vi "Proceed.vi"(7 "component is ready (Y)":bool=TRUE, 8 "error in (no error)":errorcluster, 10 "ProceedMessage":refnum<class "ProceedMessage.lvclass">, 11 "DAQCascade512II in":refnum<class "DAQCascade512II.lvclass">) -> (0 "error out":errorcluster, 2 "all observers are ready?":bool, 3 "DAQCascade512II out":refnum<class "DAQCascade512II.lvclass">)   [LabVIEW 2012, in "DAQCascade512II.lvclass"]
doc: "The Proceed method is used to check if your component is ready. Also it checks if the observers are ready. When the observers and the component are ready, it sends the proceed to its observee. If it's the highest observee, it distributes a stop command."
uses:
  DAQCascade512II.lvclass
  <vilib>/Distrio/Murmex/ProceedMessage/ProceedMessage.lvclass
  DAQCascade512II.lvclass/DAQCascade512II.ctl
  <vilib>/Distrio/Murmex/StopMessage/StopMessage.lvclass
  <vilib>/Distrio/Murmex/Murmex/Murmex.lvclass
panel:
  # "This method is called when the PROCEED\ntrigger is sent. \n\nOverride this method when your component needs to\nrespond to this trigger. \n\nCall parent for proper implementation"
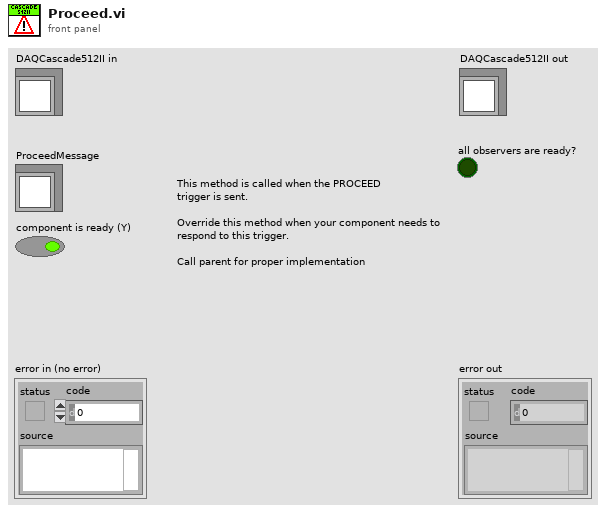
[diagram p1: front panel]
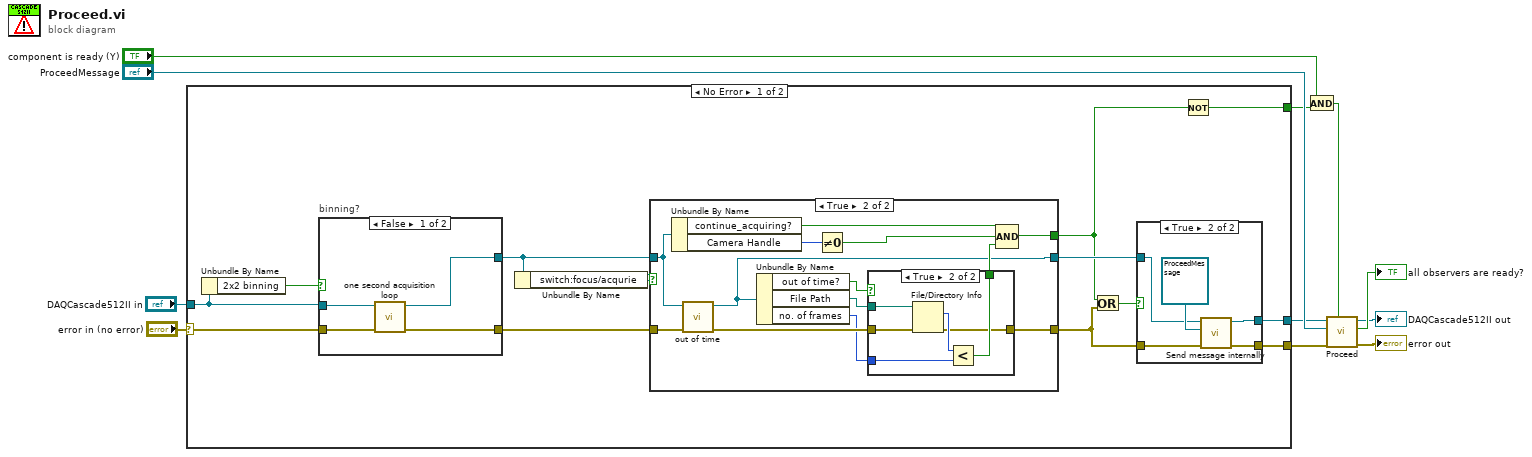
[diagram p0: block diagram]
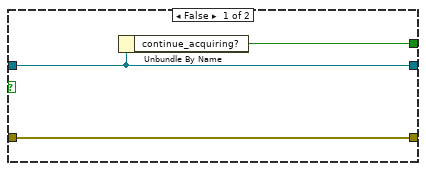
[diagram p2: hidden frame]
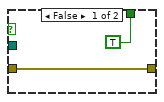
[diagram p3: hidden frame]
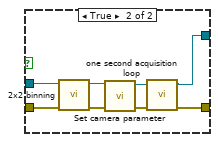
[diagram p4: hidden frame]
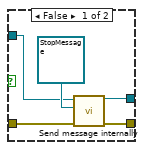
[diagram p5: hidden frame]
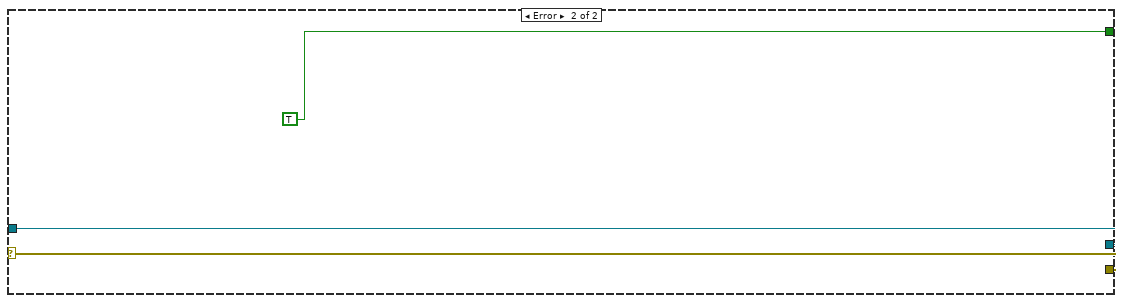
[diagram p6: hidden frame]
diagram:
  n1 = case shown="No Error" "error in (no error)" {
    selector: "error in (no error)" -> [w17 w72]
    tunnel: "DAQCascade512II in" -> [w18 w73]
    tunnel: [w24 w72] -> w5
    tunnel: [w23 w73] -> w4
    tunnel: [w16 TRUE ("continue_acquiring?")] -> w2
    frame No Error {
      n2 = Unbundle By Name(w18) -> ("2x2 binning"=w22:bool)
      n3 = case "binning?" shown="False" w22 {
        tunnel: w17 -> [w52 w59]
        tunnel: w18 -> [w49 w60]
        tunnel: [w51 w55] -> w21
        tunnel: [w50 w56] -> w19
        frame False {
          n4 = call-dynamic "one second acquisition loop.vi"("error in (no error)"=w52, "DAQCascade512II"=w49) -> ("error out"=w51:errorcluster, "DAQCascade512II out"=w50:refnum<class "DAQCascade512II.lvclass">)  [unwired: 8 in]
        }
        frame True {
          n5 = call-dynamic "2x2 binning.vi"("error in"=w59, "DAQCascade512II in"=w60) -> ("error out"=w57:errorcluster, "DAQCascade512II out"=w58:refnum<class "DAQCascade512II.lvclass">)  [unwired: 8 in]
          n6 = call-dynamic "Set camera parameter.vi"("error in (no error)"=w57, "DAQCascade512II in"=w58) -> ("error out"=w54:errorcluster, "DAQCascade512II out"=w53:refnum<class "DAQCascade512II.lvclass">)  [unwired: 8 in]
          n7 = call-dynamic "one second acquisition loop.vi"("error in (no error)"=w54, "DAQCascade512II"=w53) -> ("error out"=w55:errorcluster, "DAQCascade512II out"=w56:refnum<class "DAQCascade512II.lvclass">)  [unwired: 8 in]
        }
      }
      n8 = Unbundle By Name(w19) -> ("switch:focus/acqurie"=w12:bool)
      n9 = case shown="True" w12 {
        tunnel: [w25 w38] -> w13
        tunnel: w19 -> [w26 w36]
        tunnel: w21 -> [w27 w35]
        tunnel: [w27 w29] -> w15
        tunnel: [w26 w28] -> w20
        frame False {
          n10 = Unbundle By Name(w26) -> ("continue_acquiring?"=w25:bool)
        }
        frame True {
          n11 = Unbundle By Name(w36) -> ("continue_acquiring?"=w37:bool, "Camera Handle"=w40:u32)
          n12 = call-dynamic "out of time.vi"("error constant"=w35, "DAQCascade512II 2"=w36) -> ("error constant 2"=w32:errorcluster, "DAQCascade512II"=w28:refnum<class "DAQCascade512II.lvclass">)  [unwired: 8 in]
          n13 = Unbundle By Name(w28) -> ("out of time?"=w34:bool, "File Path"=w33:path, "no. of frames"=w31:u32)
          n14 = Not Equal To 0?(x=w40) -> (x != 0?=w39:bool)
          n15 = case shown="True" w34 {
            tunnel: w33 -> [_ w48]
            tunnel: w32 -> [w42 w47]
            tunnel: w31 -> [_ w46]
            tunnel: [TRUE w44] -> w30
            tunnel: [w42 w43] -> w29
            frame False {
            }
            frame True {
              n16 = File/Directory Info(path=w48, error in=w47) -> (size=w45:i64, error out=w43:errorcluster)  [unwired: 5 out]
              n17 = Less?(x=w45, y=w46) -> (x < y?=w44:bool)
            }
          }
          n18 = Compound Arithmetic op=AND(w37, w39, w30) -> (w38:bool)
        }
      }
      n19 = Or(x=w13, y=w15) -> (x .or. y?=w14:bool)
      n20 = case shown="True" w14 {
        tunnel: [w65 w69] -> w24
        tunnel: [w63 w68] -> w23
        tunnel: w15 -> [w61 w67]
        tunnel: w20 -> [w62 w66]
        frame False {
          n21 = call <vilib>:"Send message internally.vi"("error in (no error)"=w61, "Message"=refnum<class "StopMessage.lvclass"> refnum ("Distrio Murmex 1.5:StopMessage"), "Murmex in"=w62) -> ("error out"=w65:errorcluster, "Murmex out"=w63:refnum<class "DAQCascade512II.lvclass">)  [unwired: 7 in]
        }
        frame True {
          n22 = call <vilib>:"Send message internally.vi"("error in (no error)"=w67, "Message"=refnum<class "ProceedMessage.lvclass"> refnum ("Distrio Murmex 1.5:ProceedMessage"), "Murmex in"=w66) -> ("error out"=w69:errorcluster, "Murmex out"=w68:refnum<class "DAQCascade512II.lvclass">)  [unwired: 7 in]
        }
      }
      n23 = Not(x=w13) -> (.not. x?=w16:bool)
    }
    frame Error {
    }
  }
  n24 = And(x="component is ready (Y)", y=w2) -> (x .and. y?=w1:bool)
  n25 = call-parent "Proceed.vi"("component is ready (Y)"=w1, "error in (no error)"=w5, "ProceedMessage"="ProceedMessage", "Murmex in"=w4) -> ("error out"=→"error out":errorcluster, "all observers are ready?"=→"all observers are ready?":bool, "Murmex out"=→"DAQCascade512II out":refnum<class "DAQCascade512II.lvclass">)  [unwired: 5 in]
